vi "GetTextSize.vi"(8 "Error In":errorcluster, 9 "Text":string, 10 "Font":refnum<k24>, 11 "Graphics":refnum<k24>) -> (0 "Error Out":errorcluster, 2 "Height":sgl, 3 "Width":sgl)   [LabVIEW 2020, in "LcPictureBox.lvclass"]
uses:
  LcPictureBox.lvclass
  System.Drawing
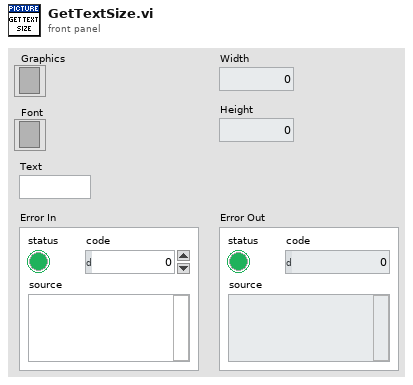
[diagram p1: front panel]
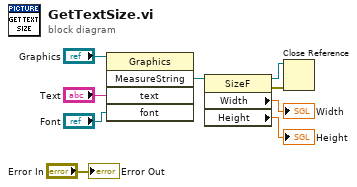
[diagram p0: block diagram]
diagram:
  n1 = invoke class="Graphics" method="MeasureString"(reference="Graphics", "text"="Text", "font"="Font") -> ("MeasureString"=w1:refnum<k24>)  [unwired: 2 in, 4 out]
  n2 = property class="SizeF"(reference=w1) -> (reference out=w3:refnum<k24>, error out=w4:errorcluster, "Width"=→"Width":sgl, "Height"=→"Height":sgl)  [unwired: 1 in]
  n3 = Close Reference(reference=w3, error in (no error)=w4) -> ()  [unwired: 1 out]
  "Error Out" <- "Error In"
